vi "PH_BL-Master.get Picture Status Service Subscriber Status by Name.vi"(0 "i ref in":refnum<vi>, 2 "Picture Status Subscriber Instance":string="N/A", 5 "error in (no error)":errorcluster) -> (9 "index of element":i32, 10 "Pic GUI Ref":refnum<vi>, 11 "no Link?":bool, 13 "Instance found?":bool, 14 "i ref out":refnum<vi>, 15 "off/false/out?":bool, 16 "on/true/in?":bool, 17 "Subscriber State":T1 items=["no info", "off/false/out", "on/true/in", "Failure", "Alarm", "Status 1", "Status 2", "Status 3"], 18 "off/false/out or on/true/in?":bool, 19 "error out":errorcluster)   [LabVIEW 2014, in "PH_BL-Master.lvlib"]
doc: "This VI gets the status of the selected Subscriber."
uses:
  PH_BL-Master.lvlib
  PH_Basics/PH_StatusHandler/PH_StatusHandler.Status.ctl
  PH_Basics/PH_StatusHandler/PH_StatusHandler.lvlib
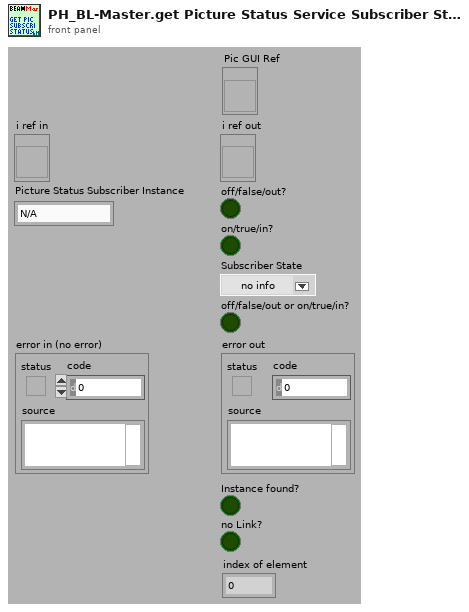
[diagram p1: front panel]
types:
  T1 = typedef "PH_StatusHandler.lvlib/PH_StatusHandler.Status.ctl" = i16
  T2 = typedef "PH_BL-Master.lvlib/PH_BL-Master.i attribute.ctl" = cluster{"Remote controlled":bool, "Boolean Condition Service Subscriber":refnum<vi>[], "Picture Condition Service Subscriber":refnum<vi>[], "R2S":cluster{"GUI Ref":refnum<vi>, "State":bool}, "Vacua":cluster{"GUI Ref":refnum<vi>, "Limit":dbl, "Curr Value":dbl, "in range":bool}[], "O2 Inspection":cluster{"GUI Ref":refnum<vi>, "Concentration":dbl, "State":T1}[], "Boolean Status Service Subscriber":cluster{"GUI Ref":refnum<vi>, "Status":T1, "no Link?":bool, "Status Subscriber Class":T3}[], "Picture Status Service Subscriber":cluster{"GUI Ref":refnum<vi>, "Status":T1, "no Link?":bool, "Status Subscriber Class":T3}[], "6P 4Q Service Subscriber":cluster{"GUI Ref":refnum<vi>, "Selector":T4, "no Link?":bool}[], "Index of latest 6P 4Q changing Instance":i32, "Index of latest Picture Status changing Instance":i32, "Index of latest Boolean Status changing Instance":i32, "Vision ID on same Node":string, "Start Phase over?":bool, "GUI Ref Delete":refnum<vi>}
  T3 = typedef "PH_BL-Master.lvlib/PH_BL-Master.Status Subscriber Class.ctl" = enum16{"unknown", "Switch", "BB", "6P Switch", "Switch GUI", "Switch and 6P State", "Force Sensor"}
  T4 = typedef "PH_4_Pos_Selector.lvlib/PH_4_Pos_Selector.Position Selector.ctl" = u16
  T5 = cluster{"GUI Ref":refnum<vi>, "Status":T1, "no Link?":bool, "Status Subscriber Class":T3}[]
  T6 = cluster{"GUI Ref":refnum<vi>, "Status":T1, "no Link?":bool, "Status Subscriber Class":T3}
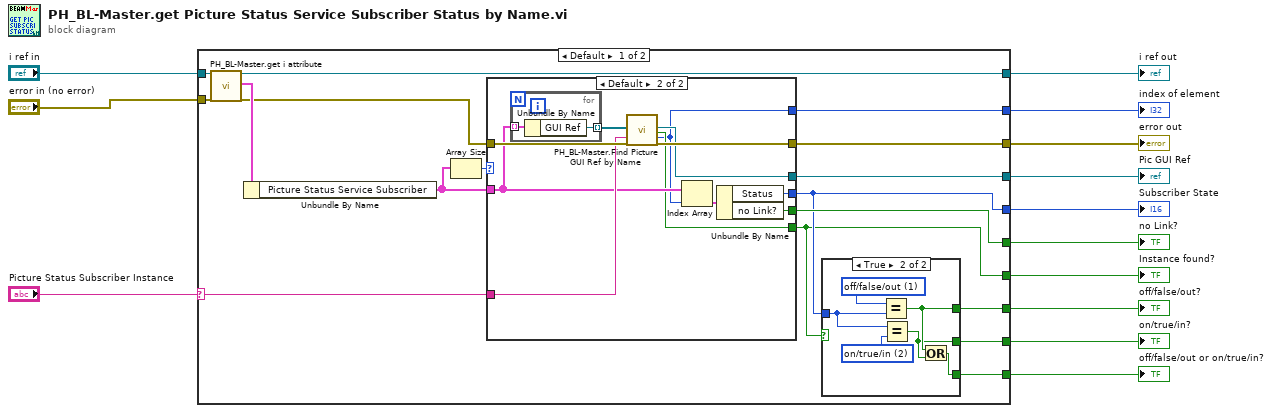
[diagram p0: block diagram]
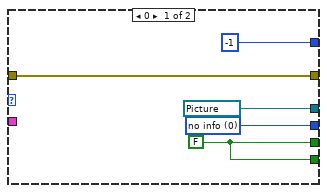
[diagram p2: hidden frame]
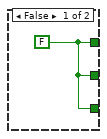
[diagram p3: hidden frame]
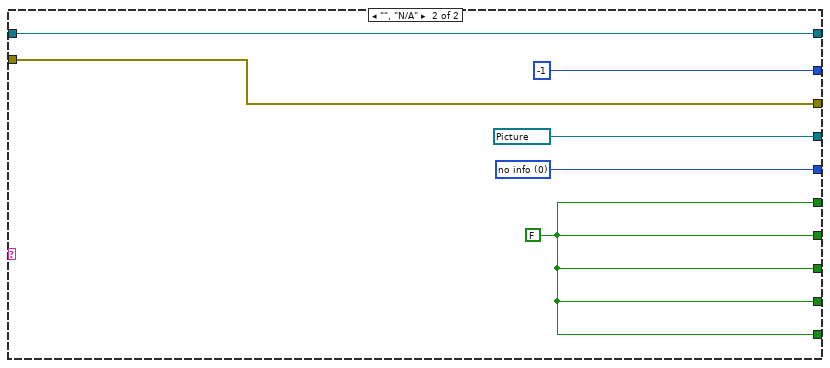
[diagram p4: hidden frame]
diagram:
  n1 = case shown="Default" "Picture Status Subscriber Instance" {
    selector: "Picture Status Subscriber Instance" -> [w24 _]
    tunnel: "error in (no error)" -> [w29 w60]
    tunnel: "i ref in" -> [w28 w61]
    tunnel: [w27 w61] -> w5
    tunnel: [w17 w59] -> w7
    tunnel: [w26 w60] -> w6
    tunnel: [w21 w58] -> w8
    tunnel: [w20 w58] -> w9
    tunnel: [w19 w58] -> w10
    tunnel: [w14 w58] -> w4
    tunnel: [w25 w58] -> w3
    tunnel: [w22 refnum<vi> refnum ("Wanted Pic GUI Ref")] -> w2
    tunnel: [w18 -1 ("index of element")] -> w1
    frame Default {
      n2 = call "PH_BL-Master.get i attribute.vi"("i ref in"=w28, "error in (no error)"=w29) -> ("i ref out"=w27:refnum<vi>, "i attribute"=w30:T2, "error out"=w16:errorcluster)  [unwired: 15 in]
      n3 = Unbundle By Name(w30) -> ("Picture Status Service Subscriber"=w23:T5)
      n4 = Array Size(array=w23) -> (size(s)=w15:i32)
      n5 = case shown="Default" w15 {
        tunnel: w23 -> [_ w42]
        tunnel: w24 -> [_ w44]
        tunnel: [w35 w43] -> w26
        tunnel: [w34 w39] -> w17
        tunnel: w16 -> [w35 w45]
        tunnel: [w33 w38] -> w14
        tunnel: [w33 w40] -> w25
        tunnel: [refnum<vi> refnum ("Wanted Pic GUI Ref") w37] -> w22
        tunnel: [-1 ("index of element") w36] -> w18
        frame 0 {
          w33 = FALSE
          w34 = T1 0 items=["no info", "off/false/out", "on/true/in", "Failure", "Alarm", "Status 1", "Status 2", "Status 3"] ("State")
        }
        frame Default {
          n6 = for {
            tunnel: w42 -> [w48] mode=indexing
            tunnel: [w47] -> w46 mode=indexing
            n7 = Unbundle By Name(w48) -> ("GUI Ref"=w47:refnum<vi>)
          }
          n8 = call "PH_BL-Master.Find Picture GUI Ref by Name.vi"("Pic Ref Array"=w46, "Label"=w44, "error in"=w45) -> ("Wanted Pic GUI Ref"=w37:refnum<vi>, "Ref found?"=w38:bool, "index of element"=w36:i32, "error out"=w43:errorcluster)  [unwired: 13 in]
          n9 = Index Array(array=w42, index=w36) -> (element=w41:T6)
          n10 = Unbundle By Name(w41) -> ("Status"=w39:T1, "no Link?"=w40:bool)
        }
      }
      n11 = case shown="True" w14 {
        tunnel: [w49 w54] -> w21
        tunnel: [w49 w53] -> w20
        tunnel: [w49 w52] -> w19
        tunnel: w17 -> [_ w50]
        frame False {
          w49 = FALSE
        }
        frame True {
          w55 = T1 2 items=["no info", "off/false/out", "on/true/in", "Failure", "Alarm", "Status 1", "Status 2", "Status 3"] ("y")
          w51 = T1 1 items=["no info", "off/false/out", "on/true/in", "Failure", "Alarm", "Status 1", "Status 2", "Status 3"] ("y")
          n12 = Equal?(x=w51, y=w50) -> (x = y?=w54:bool)
          n13 = Equal?(x=w50, y=w55) -> (x = y?=w53:bool)
          n14 = Or(x=w54, y=w53) -> (x .or. y?=w52:bool)
        }
      }
    }
    frame "", "N/A" {
      w58 = FALSE
      w59 = T1 0 items=["no info", "off/false/out", "on/true/in", "Failure", "Alarm", "Status 1", "Status 2", "Status 3"] ("State")
    }
  }
  "i ref out" <- w5
  "error out" <- w6
  "Subscriber State" <- w7
  "off/false/out?" <- w8
  "on/true/in?" <- w9
  "off/false/out or on/true/in?" <- w10
  "Instance found?" <- w4
  "no Link?" <- w3
  "Pic GUI Ref" <- w2
  "index of element" <- w1
